vi "Update Property.vi"(8 "error in (no error)":errorcluster, 9 "Value":variant, 10 "Name":string, 11 "BooleanPanel in":refnum<class "BooleanPanel.lvclass">) -> (0 "error out":errorcluster, 3 "BooleanPanel out":refnum<class "BooleanPanel.lvclass">)   [LabVIEW 2020, in "Conditum-Tools.lvlib" / "BooleanPanel.lvclass"]
uses:
  BooleanPanel.lvclass
  BooleanPanel.lvclass/BooleanPanel.ctl
  Conditum-Clone/Columns/Boolean/Boolean.lvclass
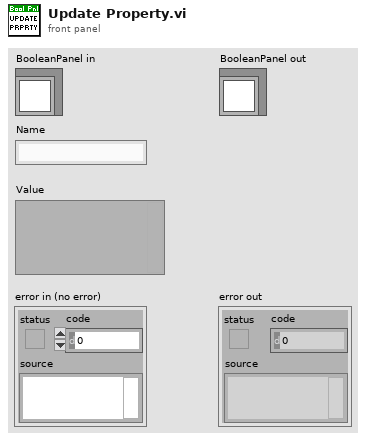
[diagram p1: front panel]
types:
  T1 = typedef "Conditu2.lvlib/Columns.lvlib/Boolean.lvclass/Definition.ctl" = cluster{"Default":bool}
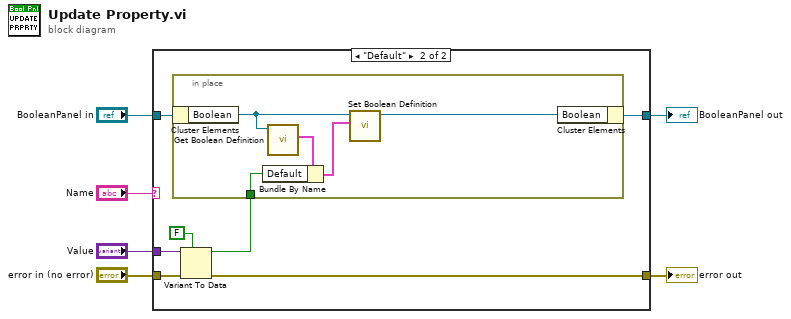
[diagram p0: block diagram]
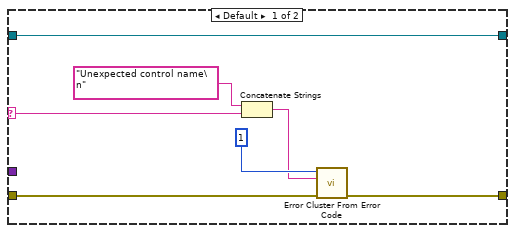
[diagram p2: hidden frame]
diagram:
  n1 = case shown="\"Default\"" "Name" {
    selector: "Name" -> [w9 _]
    tunnel: "Value" -> [_ w20]
    tunnel: "BooleanPanel in" -> [w7 w16]
    tunnel: "error in (no error)" -> [w13 w18]
    tunnel: [w12 w17] -> w2
    tunnel: [w7 w14] -> w1
    frame Default {
      n2 = Concatenate Strings("Unexpected control name\n" ("format string"), w9) -> (w8:string)
      n3 = call <vilib>:"Error Cluster From Error Code.vi"("error in (no error)"=w13, "error message (\"\")"=w8, "error code (0)"=1) -> ("error out"=w12:errorcluster)  [unwired: 6 in]
    }
    frame "Default" {
      n4 = Variant To Data(error in=w18, type=FALSE, Variant=w20) -> (data=w15:bool, error out=w17:errorcluster)
      n5 = in-place {
        in-place-border: w15 -> [w24]
        n6 = in-place-cluster #1(w16) -> ("Boolean"=w23:refnum<class "Boolean.lvclass">)
        n7 = call "Get Boolean Definition.vi"("Boolean in"=w23) -> ("Definition"=w25:T1)  [unwired: 10 in]
        n8 = Bundle By Name(cluster=w25, "Default"=w24) -> (w22:T1)
        n9 = call "Set Boolean Definition.vi"("Boolean Definition"=w22, "Boolean in"=w23) -> ("Boolean out"=w21:refnum<class "Boolean.lvclass">)  [unwired: 9 in]
        n10 = in-place-cluster #1("Boolean"=w21) -> (w14:refnum<class "BooleanPanel.lvclass">)
      }
    }
  }
  "error out" <- w2
  "BooleanPanel out" <- w1
